vi "Camera Final.vi"(11 "Image Src":T1) -> (0 "Image Dst Out 2":T1(plugin-control), 1 "Can Fit":bool, 2 "Viable Image":bool, 3 "Can Hit":bool, 4 "Possible Velocity":bool, 5 "Velocity":dbl, 6 "Centered":bool)   [LabVIEW 2015]
uses:
  <vilib>/vision/Image Controls.llb/IMAQ Image.ctl
  <vilib>/vision/NI_Vision_Development_Module.lvlib
panel:
  out "Center of Mass.X":dbl
  out "Width inches":dbl
  out "Distance":dbl
  out "Height":dbl
  out "Width":dbl
  out "element":T2
  out "Array":cluster{dbl, i32}[](array[cluster])
  out "Image Dst Out":T1(plugin-control)
  out "Particle Reports (Pixels)":T3(array[cluster]) {"Orientation" format="%.2f"; "Dimensions"."Height" format="%.2f"; "Dimensions"."Width" format="%.2f"; "Center of Mass"."Y" format="%.2f"; "Center of Mass"."X" format="%.2f"; "Bounding Rect"."Bottom" format="%.2f"; "Bounding Rect"."Right" format="%.2f"; "Bounding Rect"."Top" format="%.2f"; "Bounding Rect"."Left" format="%.2f"; "Number of Holes" format="%.2f"; "Area" format="%.2f"}
  out "Number of Particles":i32
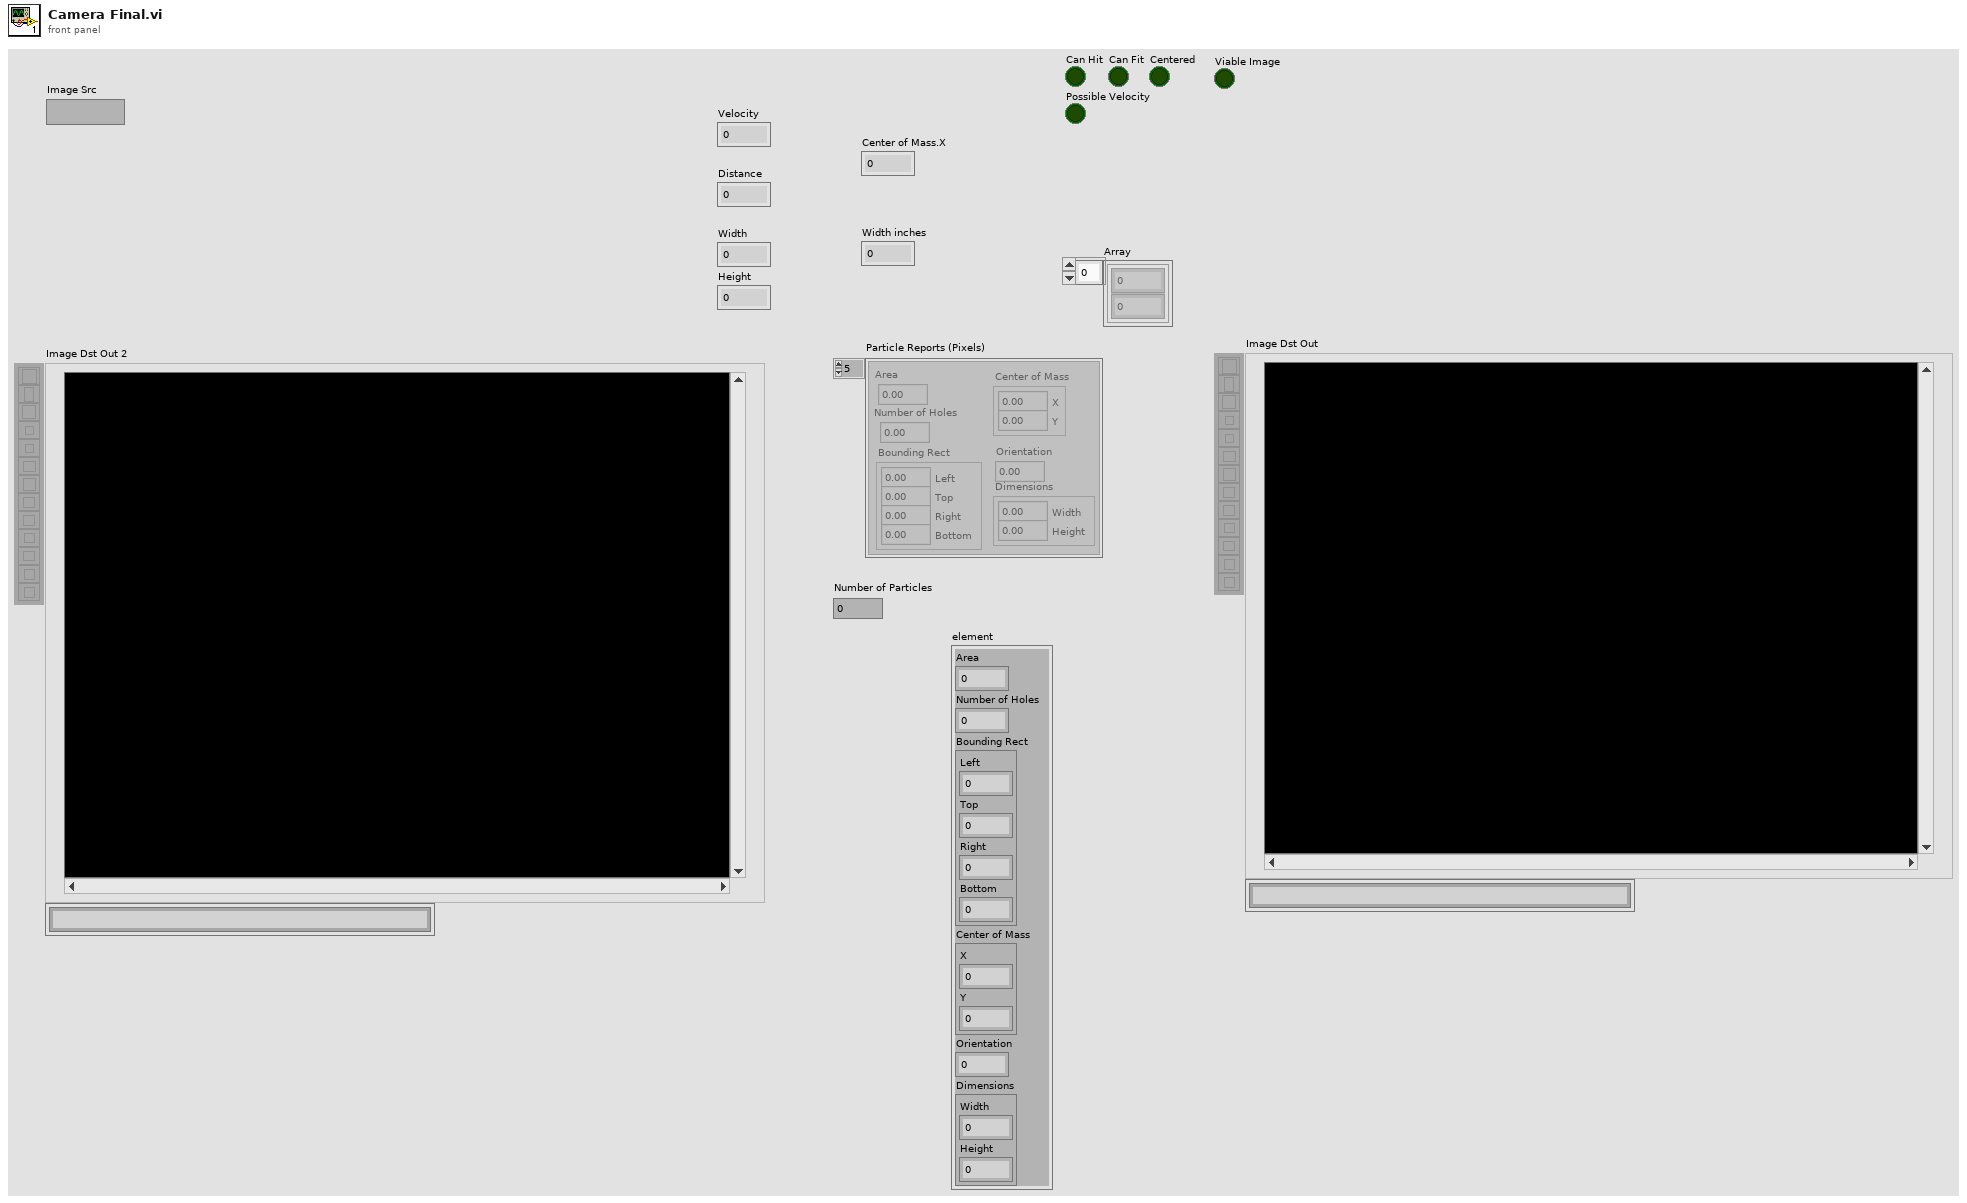
[diagram p1: front panel]
types:
  T1 = typedef "IMAQ Image.ctl" = refnum<image>
  T2 = cluster{"Area":dbl, "Number of Holes":dbl, "Bounding Rect":cluster{"Left":dbl, "Top":dbl, "Right":dbl, "Bottom":dbl}, "Center of Mass":cluster{"X":dbl, "Y":dbl}, "Orientation":dbl, "Dimensions":cluster{"Width":dbl, "Height":dbl}}
  T3 = cluster{"Area":dbl, "Number of Holes":dbl, "Bounding Rect":cluster{"Left":dbl, "Top":dbl, "Right":dbl, "Bottom":dbl}, "Center of Mass":cluster{"X":dbl, "Y":dbl}, "Orientation":dbl, "Dimensions":cluster{"Width":dbl, "Height":dbl}}[]
  T4 = cluster{"Brightness":sgl, "Contrast":sgl, "Gamma":sgl}
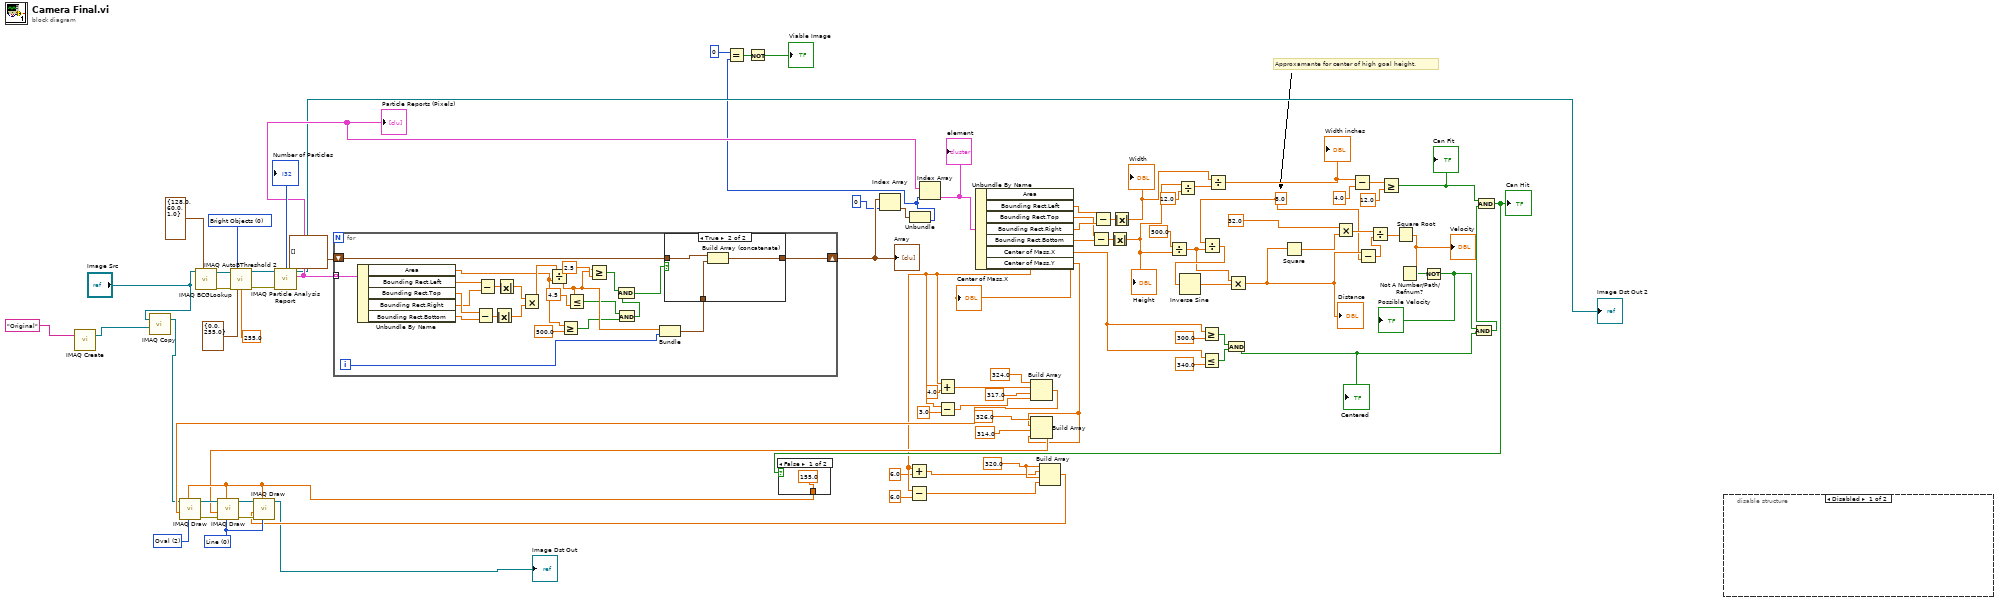
[diagram p0: block diagram]
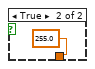
[diagram p3: hidden frame]
diagram:
  w9 = 8.0 ("x")
  w20 = 320.0 ("element")
  w33 = u16 0 items=["Line", "Rectangle", "Oval"] ("Shape to draw")
  w39 = u16 2 items=["Line", "Rectangle", "Oval"] ("Shape to draw")
  w76 = u32 0 items=["Bright Objects", "Dark Objects"] ("Look For (Bright Objects)")
  # "Approxamante for center of high goal height."
  n1 = call "IMAQ Create"("Image Name"="Original") -> ("New Image"=w78:T1)  [unwired: 4 in, 1 out]
  n2 = call "IMAQ Copy"("Image Dst"=w78, "Image Src"="Image Src") -> ("Image Dst Out"=w7:T1)  [unwired: 4 in, 1 out]
  n3 = call "IMAQ BCGLookup"("Image Src"="Image Src", "BCG Values"=T4 {"Brightness"=128.0, "Contrast"=60.0, "Gamma"=1.0}) -> ("Image Dst Out"=w84:T1, "error out"=w83:errorcluster)  [unwired: 5 in]
  n4 = call "IMAQ AutoBThreshold 2"("Image Src"=w84, "Look For (Bright Objects)"=w76, "error in (no error)"=w83, "Threshold Limits"=cluster{"Lower value":sgl, "Upper value":sgl} {"Lower value"=0.0, "Upper value"=255.0}, "Replace Value (1)"=sgl 255.0) -> ("Image Dst Out"=w81:T1, "error out"=w80:errorcluster)  [unwired: 8 in, 1 out]
  n5 = call "IMAQ Particle Analysis Report"("error in (no error)"=w80, "Image"=w81) -> ("Particle Reports (Pixels)"=w74:T3, "Image Out (duplicate)"=→"Image Dst Out 2":T1, "Number of Particles"=→"Number of Particles":i32)  [unwired: 4 in, 3 out]
  "Particle Reports (Pixels)" <- w74
  n6 = for {
    tunnel: w74 -> [w110] mode=indexing
    shift-right: [w98] -> w72
    shift-left: cluster{dbl, i32}[] [] -> [w97]
    i -> [w100]
    n7 = Unbundle By Name(w110) -> ("Area"=w93:dbl, "Bounding Rect.Left"=w106:dbl, "Bounding Rect.Top"=w108:dbl, "Bounding Rect.Right"=w107:dbl, "Bounding Rect.Bottom"=w109:dbl)
    n8 = Subtract(x=w108, y=w109) -> (x-y=w104:dbl)
    n9 = Subtract(x=w106, y=w107) -> (x-y=w105:dbl)
    n10 = Absolute Value(x=w104) -> (abs(x)=w102:dbl)
    n11 = Absolute Value(x=w105) -> (abs(x)=w103:dbl)
    n12 = Multiply(x=w103, y=w102) -> (x*y=w101:dbl)
    n13 = Divide(x=w101, y=w93) -> (x/y=w92:dbl)
    n14 = Greater Or Equal?(x=w93, y=500.0) -> (x >= y?=w91:bool)
    n15 = Less Or Equal?(x=w92, y=4.5) -> (x <= y?=w90:bool)
    n16 = Greater Or Equal?(x=w92, y=2.5) -> (x >= y?=w88:bool)
    n17 = And(x=w90, y=w91) -> (x .and. y?=w89:bool)
    n18 = And(x=w88, y=w89) -> (x .and. y?=w87:bool)
    n19 = Bundle(w92, w100) -> (w99:cluster{dbl, i32})  [unwired: 1 in]
    n20 = case shown="True" w87 {
      tunnel: w99 -> [_ w114]
      tunnel: [w111 w113] -> w98
      tunnel: w97 -> [w111 w112]
      frame False {
      }
      frame True {
        n21 = Build Array (concatenate)(w112, w114) -> (w113:cluster{dbl, i32}[])
      }
    }
  }
  "Array" <- w72
  n22 = Index Array(array=w72, index=0) -> (element=w71:cluster{dbl, i32})
  n23 = Unbundle(w71) -> (w5:i32)  [unwired: 1 out]
  n24 = Equal?(x=0, y=w5) -> (x = y?=w3:bool)
  n25 = Not(x=w3) -> (.not. x?=→"Viable Image":bool)
  n26 = Index Array(array=w74, index=w5) -> (element=w73:T2)
  "element" <- w73
  n27 = Unbundle By Name(w73) -> ("Bounding Rect.Left"=w67:dbl, "Bounding Rect.Top"=w65:dbl, "Bounding Rect.Right"=w66:dbl, "Bounding Rect.Bottom"=w64:dbl, "Center of Mass.X"=w26:dbl, "Center of Mass.Y"=w19:dbl)  [unwired: 1 out]
  "Center of Mass.X" <- w26
  n28 = Add(x=w19, y=6.0) -> (x+y=w16:dbl)
  n29 = Subtract(x=w19, y=6.0) -> (x-y=w17:dbl)
  n30 = Add(x=w19, y=4.0) -> (x+y=w31:dbl)
  n31 = Subtract(x=w19, y=3.0) -> (x-y=w30:dbl)
  n32 = Build Array(324.0 ("element"), w31, 317.0 ("element"), w30) -> (w27:dbl[])
  n33 = Build Array(326.0 ("element"), w19, 314.0 ("element"), w19) -> (w22:dbl[])
  n34 = Build Array(w20, w16, w20, w17) -> (w15:dbl[])
  n35 = Subtract(x=w65, y=w64) -> (x-y=w69:dbl)
  n36 = Subtract(x=w67, y=w66) -> (x-y=w68:dbl)
  n37 = Absolute Value(x=w69) -> (abs(x)=w57:dbl)
  "Height" <- w57
  n38 = Absolute Value(x=w68) -> (abs(x)=w54:dbl)
  "Width" <- w54
  n39 = Divide(x=500.0, y=w57) -> (x/y=w11:dbl)
  n40 = Divide(x=w57, y=12.0) -> (x/y=w55:dbl)
  n41 = Greater Or Equal?(x=w26, y=300.0) -> (x >= y?=w51:bool)
  n42 = Less Or Equal?(x=w26, y=340.0) -> (x <= y?=w50:bool)
  n43 = Divide(x=w9, y=w11) -> (x/y=w13:dbl)
  n44 = Inverse Sine(1:w13) -> (0:w12:dbl)
  n45 = Divide(x=w54, y=w55) -> (x/y=w53:dbl)
  "Width inches" <- w53
  n46 = And(x=w51, y=w50) -> (x .and. y?=w43:bool)
  "Centered" <- w43
  n47 = Multiply(x=w11, y=w12) -> (x*y=w10:dbl)
  "Distance" <- w10
  n48 = Square(x=w10) -> (x^2=w61:dbl)
  n49 = Multiply(x=32.0, y=w61) -> (x*y=w62:dbl)
  n50 = Subtract(x=w53, y=4.0) -> (x-y=w46:dbl)
  n51 = Subtract(x=w10, y=w9) -> (x-y=w59:dbl)
  n52 = Divide(x=w62, y=w59) -> (x/y=w58:dbl)
  n53 = Greater Or Equal?(x=w46, y=12.0) -> (x >= y?=w40:bool)
  "Can Fit" <- w40
  n54 = Square Root(x=w58) -> (sqrt(x)=w47:dbl)
  "Velocity" <- w47
  n55 = Not A Number/Path/Refnum?(number/path/refnum=w47) -> (NaN/Path/Refnum?=w44:bool)
  n56 = Not(x=w44) -> (.not. x?=w42:bool)
  "Possible Velocity" <- w42
  n57 = And(x=w42, y=w43) -> (x .and. y?=w41:bool)
  n58 = And(x=w40, y=w41) -> (x .and. y?=w36:bool)
  "Can Hit" <- w36
  n59 = case shown="False" w36 {
    tunnel: [sgl 155.0 ("Pixel Color") sgl 255.0 ("Pixel Color")] -> w25
    frame False {
    }
    frame True {
    }
  }
  n60 = call "IMAQ Draw"("Shape to draw"=w39, "Pixel Color"=w25, "Coordinates"=w27, "Image Src"=w7) -> ("error out"=w37:errorcluster, "Image Dst Out"=w38:T1)  [unwired: 6 in]
  n61 = call "IMAQ Draw"("Shape to draw"=w33, "Pixel Color"=w25, "error in (no error)"=w37, "Coordinates"=w22, "Image Src"=w38) -> ("error out"=w35:errorcluster, "Image Dst Out"=w34:T1)  [unwired: 5 in]
  n62 = call "IMAQ Draw"("Shape to draw"=w33, "Pixel Color"=w25, "error in (no error)"=w35, "Coordinates"=w15, "Image Src"=w34) -> ("Image Dst Out"=→"Image Dst Out":T1)  [unwired: 5 in, 1 out]
  n63 = disable-structure shown="Disabled" {
    frame Disabled {
    }
    frame Enabled {
    }
  }
